vi "Teleop.vi"(0 "Call Context":T9) -> (6 "SubState 3":T4, 9 "SubState 4":T8, 11 "Loop 3 Data":T3, 14 "SubState 0":T4=enum."driver control", 15 "Loop 1 Data":T6, 16 "Loop 0 Data":T7, 17 "SubState 1":T4, 18 "Loop 2 Data":T5, 19 "SubState 2":T4)   [LabVIEW 2013]
uses:
  typedefs/State Machine/subStates.ctl
  <vilib>/Rock Robotics/WPI/DriverStation/WPI_DriverStationDerivedRobotMode.ctl
  typedefs/State Machine/singleUseSubstate.ctl
  typedefs/Loop Datatypes/Loop 0 Datatype.ctl
  typedefs/Loop Datatypes/Loop 1 Datatype.ctl
  typedefs/Loop Datatypes/Loop 2 Datatype.ctl
  typedefs/Loop Datatypes/Loop 3 Datatype.ctl
  <vilib>/Rock Robotics/WPI/Joystick/WPI_JoystickDevRef.ctl
  <vilib>/Rock Robotics/WPI/Joystick/WPI_JoystickDeviceEnum.ctl
  typedefs/fg_typedef.ctl
  typedefs/Vision/vision enable.ctl
  <vilib>/Rock Robotics/WPI/Joystick/WPI_JoystickGetSetRefNum.vi
panel:
  out "FDC":bool
  out "JS3":T1
  out "Drive to DC":bool
  out "JS1":T1
  out "JS2":T1
  out "Exit Value":i32=-1
  # "Loop Data and Substates"
  # "Drive Loop"
  # "State Machine Master Loop"
  # "Pickup/Passing Belts Loop"
  # "Pickup/Passing Arm Loop"
  # "Pneumatics Loop"
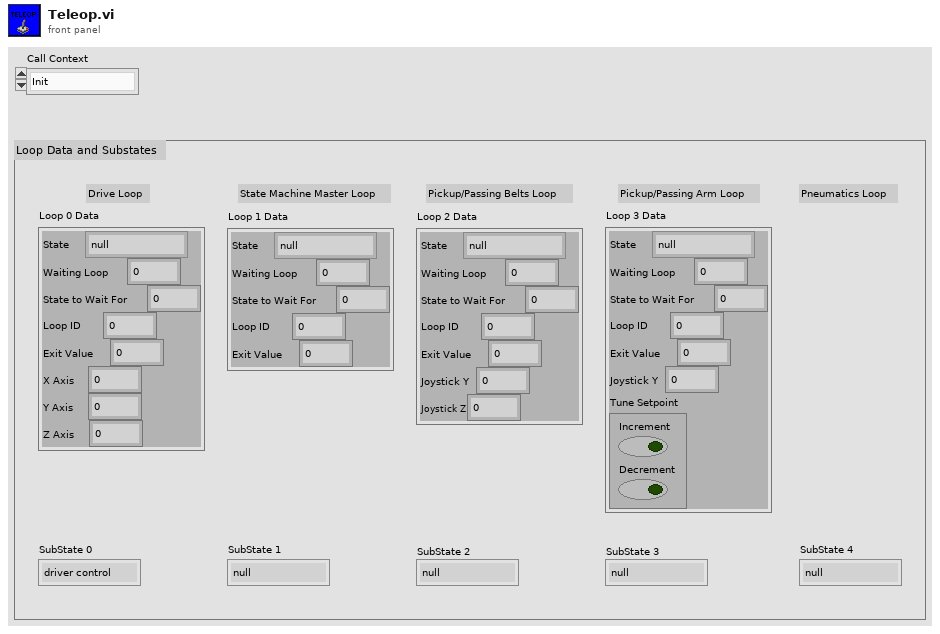
[diagram p1: front panel]
types:
  T1 = typedef "WPI_JoystickDevRef.ctl" = cluster{"Device":T2}
  T2 = typedef "WPI_JoystickDeviceEnum.ctl" = enum16{"USB 1", "USB 2", "USB 3", "USB 4", "Kinect 1", "Kinect 2"}
  T3 = typedef "Loop 3 Datatype.ctl" = cluster{"State":T4, "Waiting Loop":i32, "State to Wait For":i32, "Loop ID":i32, "Exit Value":i32, "Joystick Y":dbl, "Tune Setpoint":cluster{"Increment":bool, "Decrement":bool}}
  T4 = typedef "subStates.ctl" = enum16{"null", "wait", "driver control", "auto", "manual override", "hold position", "rotate", "pickup", "pass", "recover pass", "load", "goto shoot", "shoot high goal", "shoot low goal", "cancel arm", "cancel shooter", "end", "test"}
  T5 = typedef "Loop 2 Datatype.ctl" = cluster{"State":T4, "Waiting Loop":i32, "State to Wait For":i32, "Loop ID":i32, "Exit Value":i32, "Joystick Y":dbl, "Joystick Z":dbl}
  T6 = typedef "Loop 1 Datatype.ctl" = cluster{"State":T4, "Waiting Loop":i32, "State to Wait For":i32, "Loop ID":i32, "Exit Value":i32}
  T7 = typedef "Loop 0 Datatype.ctl" = cluster{"State":T4, "Waiting Loop":i32, "State to Wait For":i32, "Loop ID":i32, "Exit Value":i32, "X Axis":dbl, "Y Axis":dbl, "Z Axis":dbl}
  T8 = typedef "singleUseSubstate.ctl" = enum16{"null", "wait", "shift high", "shift low", "extend shooter", "retract shooter", "latch", "unlatch", "end"}
  T9 = typedef "WPI_DriverStationDerivedRobotMode.ctl" = enum16{"Init", "Execute", "Stop"}
  T10 = typedef "fg_typedef.ctl" = enum16{"Get", "Set"}
  T11 = cluster{"axis 1 (x)":dbl, "axis 2 (y)":dbl, "axis 3 (throttle)":dbl, "axis 4":dbl, "axis 5":dbl, "axis 6":dbl}
  T12 = typedef "WPI_EncoderDevRef.ctl" = cluster{"DevStatus":errorcluster, "EncoderIndex":T13, "CounterIndex":T14, "DistancePerCount":dbl, "Decoding Type":T15}
  T13 = typedef "FPGA_EncoderIdx.ctl" = enum8{"Enc 0", "Enc 1", "Enc 2", "Enc 3", "Invalid"}
  T14 = typedef "FPGA_CounterCtrSystemIndex.ctl" = enum8{"Ctr 0", "Ctr 1", "Ctr 2", "Ctr 3", "Ctr 4", "Ctr 5", "Ctr 6", "Ctr 7", "Invalid"}
  T15 = typedef "WPI_EncoderType.ctl" = enum16{"1x", "2x", "4x"}
  T16 = typedef "vision enable.ctl" = enum16{"Enable", "Disable", "Stop"}
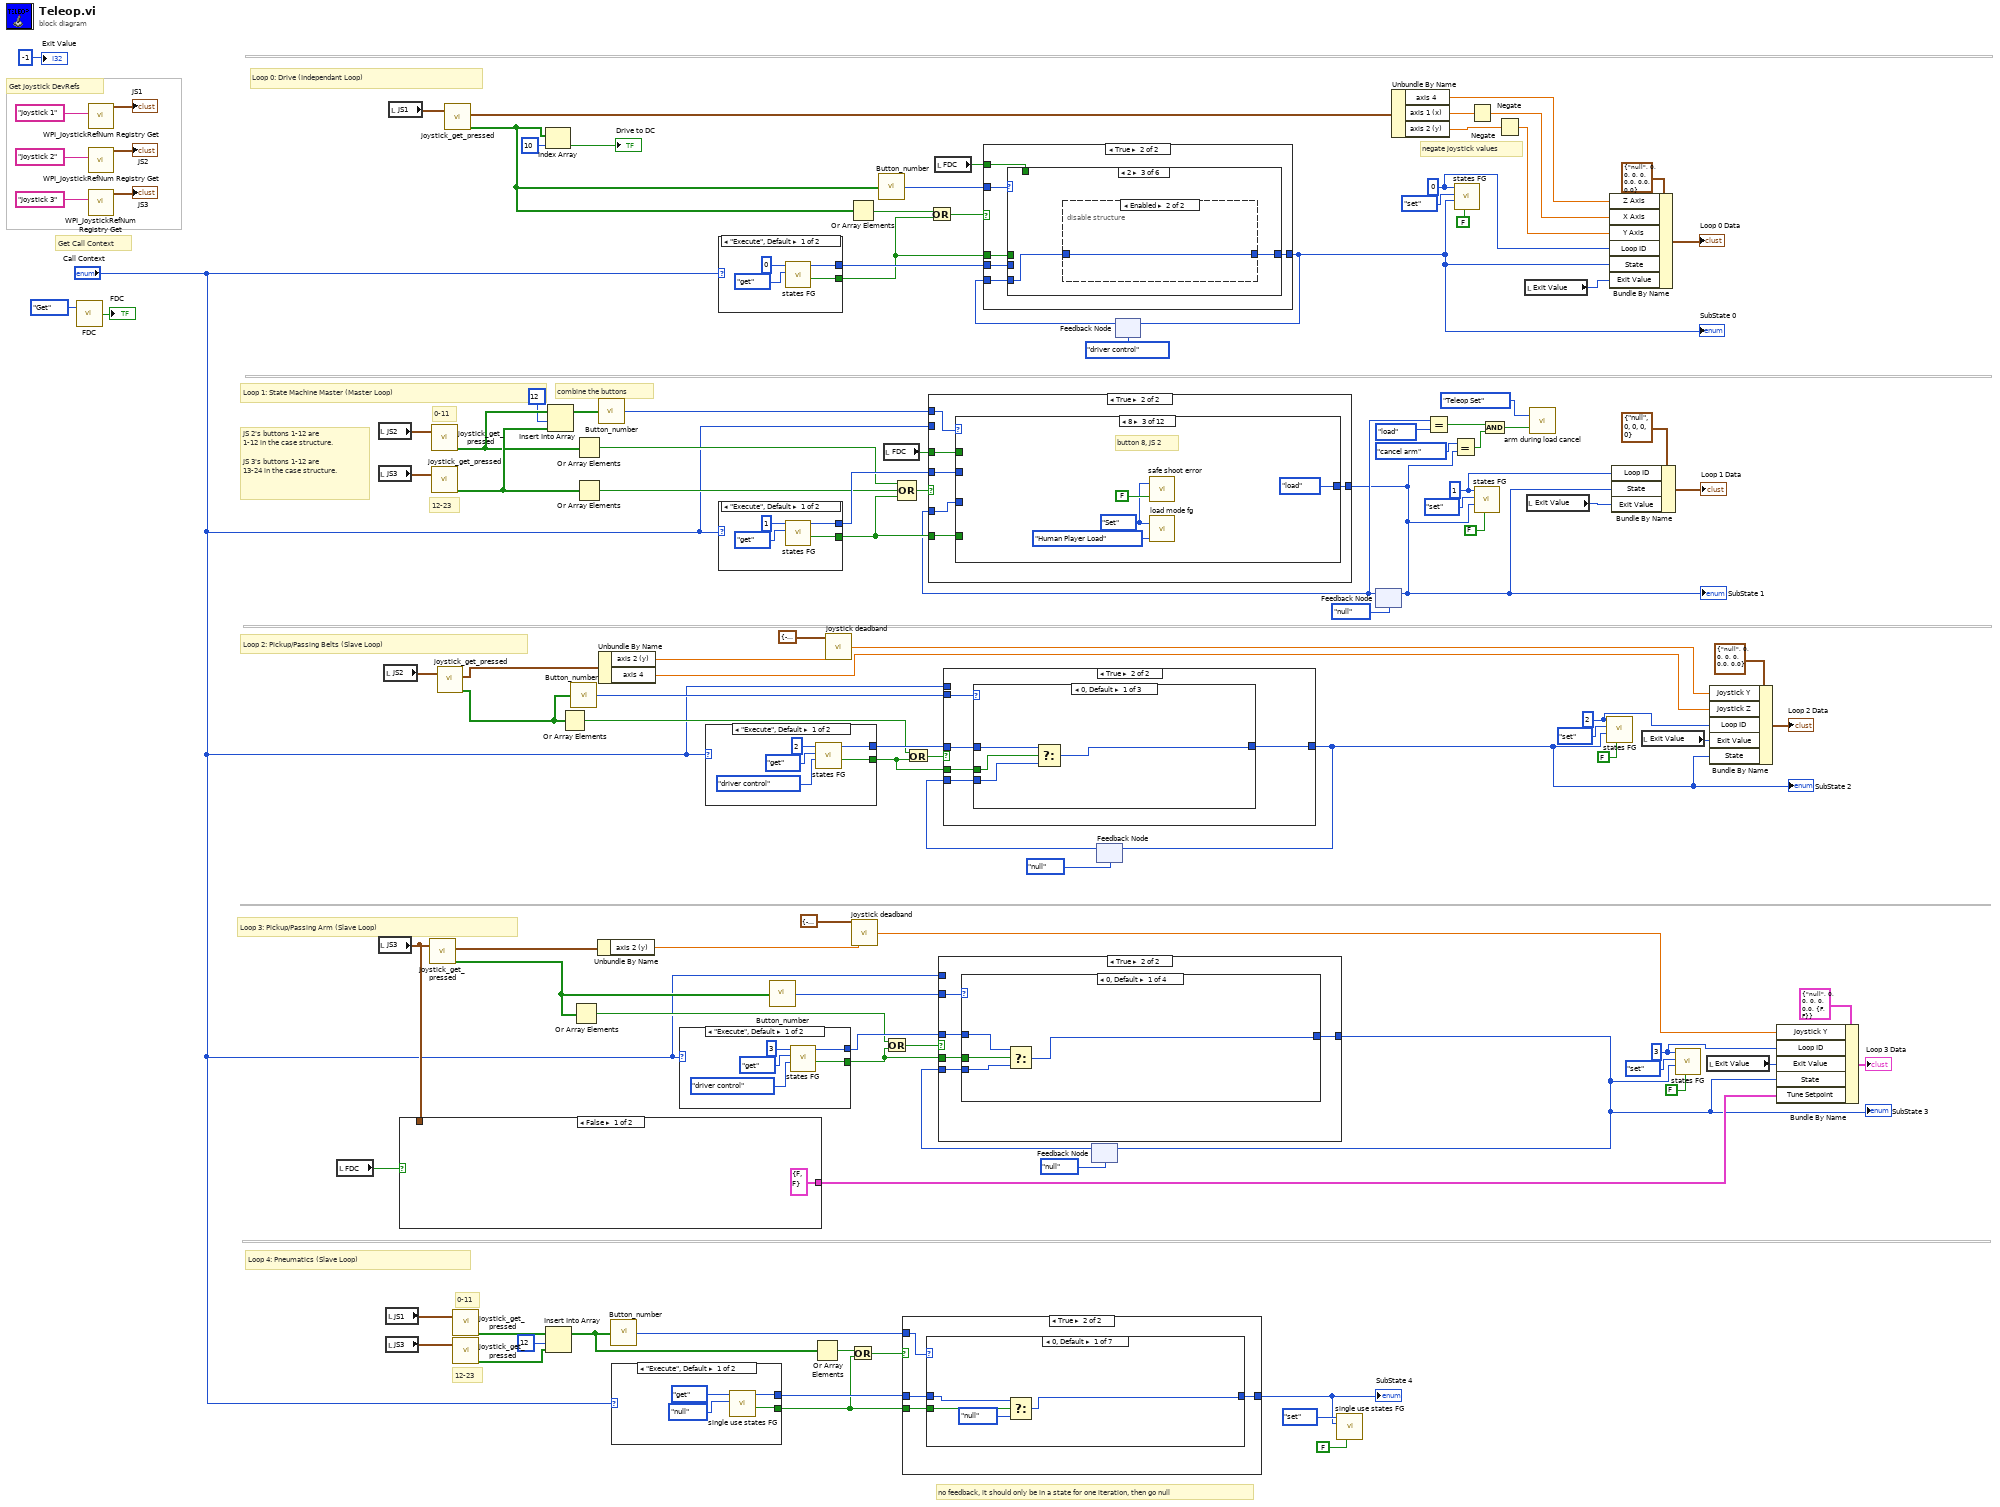
[diagram p0: block diagram]
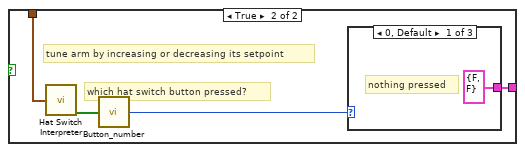
[diagram p2: hidden frame]
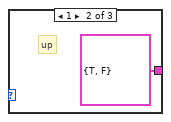
[diagram p3: hidden frame]
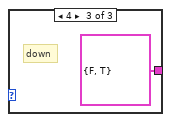
[diagram p4: hidden frame]
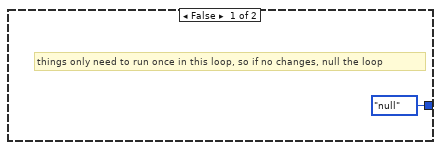
[diagram p5: hidden frame]
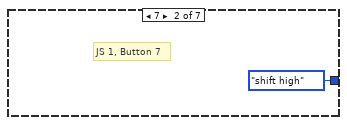
[diagram p6: hidden frame]
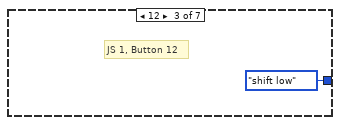
[diagram p7: hidden frame]
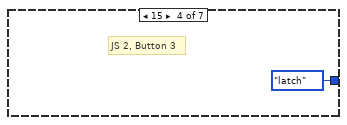
[diagram p8: hidden frame]
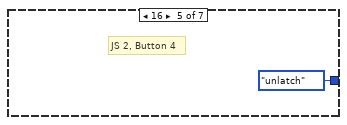
[diagram p9: hidden frame]
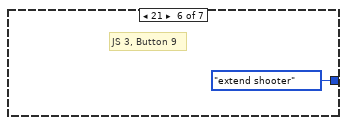
[diagram p10: hidden frame]
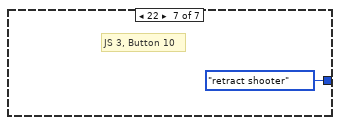
[diagram p11: hidden frame]
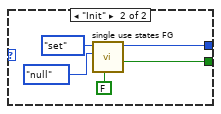
[diagram p12: hidden frame]
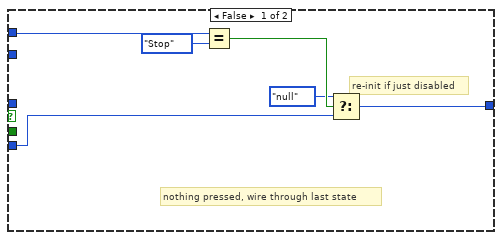
[diagram p13: hidden frame]
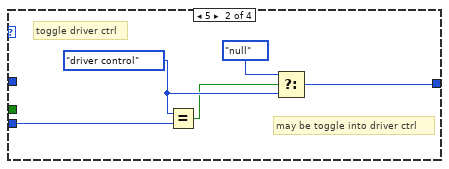
[diagram p14: hidden frame]
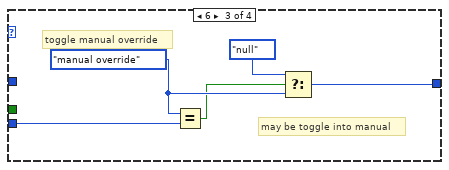
[diagram p15: hidden frame]
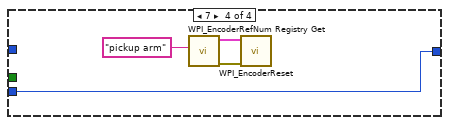
[diagram p16: hidden frame]
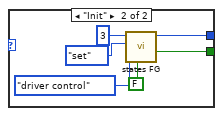
[diagram p17: hidden frame]
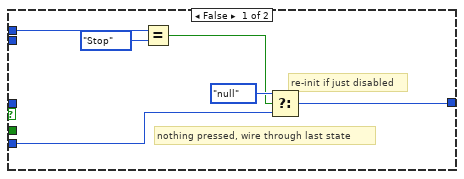
[diagram p18: hidden frame]
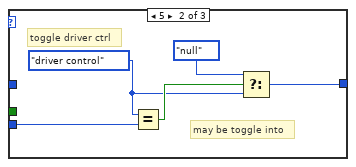
[diagram p19: hidden frame]
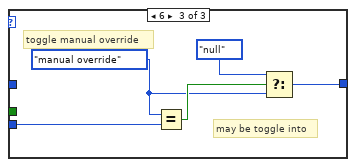
[diagram p20: hidden frame]
diagram:
  w93 = 3 ("Loop ID")
  w94 = 2 ("Loop ID")
  w103 = 1 ("Loop ID")
  w105 = 0 ("Loop ID")
  # "12-23"
  # "0-11"
  # "no feedback, it should only be in a state for one iteration, then go null"
  # "JS 2's buttons 1-12 are\n1-12 in the case structure.\n\nJS 3's buttons 1-12 are\n13-24 in the case structure."
  # "combine the buttons"
  # "12-23"
  # "0-11"
  # "negate joystick values"
  # "Get Call Context"
  # "Get Joystick DevRefs"
  # "Loop 3: Pickup/Passing Arm (Slave Loop)"
  # "Loop 4: Pneumatics (Slave Loop)"
  # "Loop 2: Pickup/Passing Belts (Slave Loop)"
  # "Loop 1: State Machine Master (Master Loop)"
  # "Loop 0: Drive (Independant Loop)"
  n1 = call "FDC.vi"("Menu"=fg_typedef."Get") -> ("FDC"=→"FDC":bool)  [unwired: 1 in]
  n2 = call <vilib>:"WPI_JoystickRefNum Registry Get.vi"("refnum name"="Joystick 1") -> ("JoystickDevRef"=→"JS1":T1)  [unwired: 9 in, 1 out]
  n3 = call <vilib>:"WPI_JoystickRefNum Registry Get.vi"("refnum name"="Joystick 2") -> ("JoystickDevRef"=→"JS2":T1)  [unwired: 9 in, 1 out]
  n4 = call <vilib>:"WPI_JoystickRefNum Registry Get.vi"("refnum name"="Joystick 3") -> ("JoystickDevRef"=→"JS3":T1)  [unwired: 9 in, 1 out]
  n5 = local read "FDC"() -> (w1:bool)
  n6 = local read "JS2"() -> (w73:T1)
  n7 = local read "JS3"() -> (w31:T1)
  n8 = local read "JS3"() -> (w40:T1)
  n9 = local read "JS2"() -> (w51:T1)
  n10 = local read "JS1"() -> (w54:T1)
  n11 = local read "JS3"() -> (w16:T1)
  n12 = local read "JS1"() -> (w74:T1)
  n13 = case shown="False" w1 {
    tunnel: w40 -> [_ w125]
    tunnel: [cluster{"Increment":bool, "Decrement":bool} {"Increment"=FALSE, "Decrement"=FALSE} w122] -> w38
    frame False {
    }
    frame True {
      # "tune arm by increasing or decreasing its setpoint"
      # "which hat switch button pressed?"
      n14 = call "Hat Switch Interpreter.vi"("JoystickDevRef"=w125) -> ("Buttons"=w124:bool[])  [unwired: 4 out]
      n15 = call "Button_number.vi"("Button Array"=w124) -> ("Button Pressed"=w123:i32)
      n16 = case shown="0, Default" w123 {
        tunnel: [cluster{"Increment":bool, "Decrement":bool} {"Increment"=FALSE, "Decrement"=FALSE} cluster{"Increment":bool, "Decrement":bool} {"Increment"=TRUE, "Decrement"=FALSE} cluster{"Increment":bool, "Decrement":bool} {"Increment"=FALSE, "Decrement"=TRUE}] -> w122
        frame 0, Default {
          # "nothing pressed"
        }
        frame 1 {
          # "up"
        }
        frame 4 {
          # "down"
        }
      }
    }
  }
  n17 = call "joystick_get_pressed.vi"("JoystickDevRef 2"=w40) -> ("Axes"=w63:T11, "Buttons Pressed?"=w7:bool[])  [unwired: 1 in, 2 out]
  n18 = call "joystick_get_pressed.vi"("JoystickDevRef 2"=w73) -> ("Buttons Pressed?"=w27:bool[])  [unwired: 1 in, 3 out]
  n19 = call "joystick_get_pressed.vi"("JoystickDevRef 2"=w31) -> ("Buttons Pressed?"=w28:bool[])  [unwired: 1 in, 3 out]
  n20 = call "joystick_get_pressed.vi"("JoystickDevRef 2"=w51) -> ("Axes"=w43:T11, "Buttons Pressed?"=w8:bool[])  [unwired: 1 in, 2 out]
  n21 = call "joystick_get_pressed.vi"("JoystickDevRef 2"=w74) -> ("Axes"=w78:T11, "Buttons Pressed?"=w56:bool[])  [unwired: 1 in, 2 out]
  n22 = call "joystick_get_pressed.vi"("JoystickDevRef 2"=w54) -> ("Buttons Pressed?"=w13:bool[])  [unwired: 1 in, 3 out]
  n23 = call "joystick_get_pressed.vi"("JoystickDevRef 2"=w16) -> ("Buttons Pressed?"=w14:bool[])  [unwired: 1 in, 3 out]
  n24 = Index Array(array=w56, index=10) -> (element=→"Drive to DC":bool)
  n25 = Insert Into Array(array=w13, index=12, new element=w14) -> (w12:bool[])
  n26 = Insert Into Array(array=w27, index=12, new element=w28) -> (w25:bool[])
  n27 = Or Array Elements(Boolean array=w8) -> (logical OR=w50:bool)
  n28 = call "Button_number.vi"("Button Array"=w8) -> ("Button Pressed"=w49:i32)
  n29 = Or Array Elements(Boolean array=w7) -> (logical OR=w62:bool)
  n30 = Or Array Elements(Boolean array=w27) -> (logical OR=w30:bool)
  n31 = Or Array Elements(Boolean array=w28) -> (logical OR=w29:bool)
  n32 = Unbundle By Name(w63) -> ("axis 2 (y)"=w59:dbl)
  n33 = call "Button_number.vi"("Button Array"=w25) -> ("Button Pressed"=w67:i32)
  n34 = Unbundle By Name(w43) -> ("axis 2 (y)"=w45:dbl, "axis 4"=w41:dbl)
  n35 = call "Button_number.vi"("Button Array"=w12) -> ("Button Pressed"=w33:i32)
  n36 = case shown="\"Execute\", Default" "Call Context" {
    tunnel: [w131 w134] -> w32
    tunnel: [w132 w133] -> w44
    frame "Execute", Default {
      n37 = call "single use states FG.vi"("substate"=singleUseSubstate."null" ("Enum"), "menu (get)"=enum16{"set", "get"}."get") -> ("exit out"=w131:bool, "substate out"=w132:T8)  [unwired: 6 in, 2 out]
    }
    frame "Init" {
      n38 = call "single use states FG.vi"("exit in"=FALSE, "substate"=singleUseSubstate."null", "menu (get)"=enum16{"set", "get"}."set") -> ("exit out"=w134:bool, "substate out"=w133:T8)  [unwired: 5 in, 2 out]
    }
  }
  n39 = case shown="\"Execute\", Default" "Call Context" {
    tunnel: [w140 w146] -> w60
    tunnel: [w138 w143] -> w91
    frame "Execute", Default {
      n40 = call "states FG.vi"("subState in"=subStates."driver control", "menu (get)"=enum16{"set", "get"}."get", "Loop ID"=3) -> ("exit out"=w140:bool, "subState out"=w138:T4)  [unwired: 5 in, 2 out]
    }
    frame "Init" {
      n41 = call "states FG.vi"("exit in"=FALSE, "subState in"=subStates."driver control", "menu (get)"=enum16{"set", "get"}."set", "Loop ID"=3) -> ("exit out"=w146:bool, "subState out"=w143:T4)  [unwired: 4 in, 2 out]
    }
  }
  n42 = case shown="\"Execute\", Default" "Call Context" {
    tunnel: [w151 w157] -> w65
    tunnel: [w149 w154] -> w109
    frame "Execute", Default {
      n43 = call "states FG.vi"("subState in"=subStates."driver control", "menu (get)"=enum16{"set", "get"}."get", "Loop ID"=2) -> ("exit out"=w151:bool, "subState out"=w149:T4)  [unwired: 5 in, 2 out]
    }
    frame "Init" {
      n44 = call "states FG.vi"("exit in"=FALSE, "subState in"=subStates."driver control", "menu (get)"=enum16{"set", "get"}."set", "Loop ID"=2) -> ("exit out"=w157:bool, "subState out"=w154:T4)  [unwired: 4 in, 2 out]
    }
  }
  n45 = case shown="\"Execute\", Default" "Call Context" {
    tunnel: [w161 w166] -> w71
    tunnel: [w160 w164] -> w108
    frame "Execute", Default {
      n46 = call "states FG.vi"("menu (get)"=enum16{"set", "get"}."get", "Loop ID"=0) -> ("exit out"=w161:bool, "subState out"=w160:T4)  [unwired: 6 in, 2 out]
    }
    frame "Init" {
      n47 = call "states FG.vi"("exit in"=FALSE, "menu (get)"=enum16{"set", "get"}."set", "Loop ID"=0) -> ("exit out"=w166:bool, "subState out"=w164:T4)  [unwired: 5 in, 2 out]
    }
  }
  n48 = case shown="\"Execute\", Default" "Call Context" {
    tunnel: [w170 w175] -> w68
    tunnel: [w169 w173] -> w107
    frame "Execute", Default {
      n49 = call "states FG.vi"("menu (get)"=enum16{"set", "get"}."get", "Loop ID"=1) -> ("exit out"=w170:bool, "subState out"=w169:T4)  [unwired: 6 in, 2 out]
    }
    frame "Init" {
      n50 = call "states FG.vi"("exit in"=FALSE, "menu (get)"=enum16{"set", "get"}."set", "Loop ID"=1) -> ("exit out"=w175:bool, "subState out"=w173:T4)  [unwired: 5 in, 2 out]
    }
  }
  n51 = call "Button_number.vi"("Button Array"=w7) -> ("Button Pressed"=w61:i32)
  n52 = Or Array Elements(Boolean array=w12) -> (logical OR=w34:bool)
  n53 = call "joystick deadband.vi"("Joystick In"=w45, "Deadband Range"=cluster{"Deadband Min":dbl, "Deadband Max":dbl} {"Deadband Min"=-0.09, "Deadband Max"=0.09}) -> ("Joystick Out"=w42:dbl)  [unwired: 4 in]
  n54 = Or Array Elements(Boolean array=w56) -> (logical OR=w72:bool)
  n55 = Or(x=w34, y=w32) -> (x .or. y?=w35:bool)
  n56 = call "joystick deadband.vi"("Joystick In"=w59, "Deadband Range"=cluster{"Deadband Min":dbl, "Deadband Max":dbl} {"Deadband Min"=-0.09, "Deadband Max"=0.09}) -> ("Joystick Out"=w39:dbl)  [unwired: 4 in]
  n57 = call "Button_number.vi"("Button Array"=w56) -> ("Button Pressed"=w77:i32)
  n58 = local read "FDC"() -> (w2:bool)
  n59 = Or(x=w62, y=w60) -> (x .or. y?=w64:bool)
  n60 = Compound Arithmetic op=OR(w30, w29, w68) -> (w69:bool)
  n61 = case shown="True" w35 {
    tunnel: [singleUseSubstate."null" ("Enum") w179] -> w10
    tunnel: w44 -> [_ w180]
    tunnel: w33 -> [_ w181]
    tunnel: w32 -> [_ w182]
    frame False {
      # "things only need to run once in this loop, so if no changes, null the loop"
    }
    frame True {
      n62 = case shown="0, Default" w181 {
        tunnel: w182 -> [w186 _ _ _ _ _ _]
        tunnel: w180 -> [w185 _ _ _ _ _ _]
        tunnel: [w184 singleUseSubstate."shift high" ("Enum") singleUseSubstate."shift low" ("Enum") singleUseSubstate."latch" ("Enum") singleUseSubstate."unlatch" ("Enum") singleUseSubstate."extend shooter" ("Enum") singleUseSubstate."retract shooter" ("Enum")] -> w179
        frame 0, Default {
          n63 = Select(t=w185, s=w186, f=singleUseSubstate."null") -> (s? t:f=w184:T8)
        }
        frame 7 {
          # "JS 1, Button 7"
        }
        frame 12 {
          # "JS 1, Button 12"
        }
        frame 15 {
          # "JS 2, Button 3"
        }
        frame 16 {
          # "JS 2, Button 4"
        }
        frame 21 {
          # "JS 3, Button 9"
        }
        frame 22 {
          # "JS 3, Button 10"
        }
      }
    }
  }
  "SubState 4" <- w10
  n64 = Or(x=w50, y=w65) -> (x .or. y?=w66:bool)
  n65 = Or(x=w72, y=w71) -> (x .or. y?=w70:bool)
  n66 = local read "FDC"() -> (w3:bool)
  n67 = feedback #1(subStates."null" ("Drive SubState")) -> (w88:T4)
  n68 = case shown="True" w64 {
    tunnel: w88 -> [w195 w199]
    tunnel: [w194 w200] -> w37
    tunnel: w91 -> [_ w201]
    tunnel: w61 -> [_ w203]
    tunnel: w60 -> [_ w202]
    tunnel: "Call Context" -> [w193 _]
    frame False {
      # "nothing pressed, wire through last state"
      # "re-init if just disabled"
      n69 = Equal?(x=w193, y=WPI_DriverStationDerivedRobotMode."Stop") -> (x = y?=w197:bool)
      n70 = Select(t=subStates."null", s=w197, f=w195) -> (s? t:f=w194:T4)
    }
    frame True {
      n71 = case shown="0, Default" w203 {
        tunnel: w202 -> [w207 _ _ _]
        tunnel: w199 -> [w206 w208 w213 w221]
        tunnel: w201 -> [w205 _ _ _]
        tunnel: [w204 w209 w214 w221] -> w200
        frame 0, Default {
          n72 = Select(t=w205, s=w207, f=w206) -> (s? t:f=w204:T4)
        }
        frame 5 {
          w211 = subStates."driver control" ("Drive SubState")
          # "may be toggle into driver ctrl"
          # "toggle driver ctrl"
          n73 = Equal?(x=w211, y=w208) -> (x = y?=w210:bool)
          n74 = Select(t=subStates."null", s=w210, f=w211) -> (s? t:f=w209:T4)
        }
        frame 6 {
          w217 = subStates."manual override" ("Drive SubState")
          # "may be toggle into manual"
          # "toggle manual override"
          n75 = Equal?(x=w217, y=w213) -> (x = y?=w215:bool)
          n76 = Select(t=subStates."null", s=w215, f=w217) -> (s? t:f=w214:T4)
        }
        frame 7 {
          n77 = call <vilib>:"WPI_EncoderRefNum Registry Get.vi"("refnum name"="pickup arm") -> ("error out"=w219:errorcluster, "EncoderDevRef"=w218:T12)  [unwired: 9 in]
          n78 = call <vilib>:"WPI_EncoderReset.vi"("error in (no error)"=w219, "EncoderDevRef"=w218) -> ()  [unwired: 8 in, 2 out]
        }
      }
    }
  }
  "SubState 3" <- w37
  n79 = feedback-in #1(w37) -> ()
  n80 = feedback #2(subStates."null" ("Drive SubState")) -> (w112:T4)
  n81 = case shown="True" w66 {
    tunnel: w112 -> [w223 w229]
    tunnel: [w222 w228] -> w36
    tunnel: w109 -> [_ w230]
    tunnel: w49 -> [_ w232]
    tunnel: w65 -> [_ w231]
    tunnel: "Call Context" -> [w224 _]
    frame False {
      # "re-init if just disabled"
      # "nothing pressed, wire through last state"
      n82 = Equal?(x=w224, y=WPI_DriverStationDerivedRobotMode."Stop") -> (x = y?=w226:bool)
      n83 = Select(t=subStates."null", s=w226, f=w223) -> (s? t:f=w222:T4)
    }
    frame True {
      n84 = case shown="0, Default" w232 {
        tunnel: w231 -> [w236 _ _]
        tunnel: w230 -> [w235 _ _]
        tunnel: w229 -> [w234 w241 w243]
        tunnel: [w233 w237 w242] -> w228
        frame 0, Default {
          n85 = Select(t=w235, s=w236, f=w234) -> (s? t:f=w233:T4)
        }
        frame 5 {
          w239 = subStates."driver control" ("Drive SubState")
          # "may be toggle into"
          # "toggle driver ctrl"
          n86 = Equal?(x=w239, y=w241) -> (x = y?=w240:bool)
          n87 = Select(t=subStates."null", s=w240, f=w239) -> (s? t:f=w237:T4)
        }
        frame 6 {
          w244 = subStates."manual override" ("Drive SubState")
          # "may be toggle into"
          # "toggle manual override"
          n88 = Equal?(x=w244, y=w243) -> (x = y?=w246:bool)
          n89 = Select(t=subStates."null", s=w246, f=w244) -> (s? t:f=w242:T4)
        }
      }
    }
  }
  "SubState 2" <- w36
  n90 = feedback-in #2(w36) -> ()
  n91 = feedback #3(subStates."driver control" ("Drive SubState")) -> (w114:T4)
  n92 = case shown="True" w70 {
    tunnel: w114 -> [w247 w250]
    tunnel: [w247 w249] -> w53
    tunnel: w108 -> [_ w251]
    tunnel: w77 -> [_ w253]
    tunnel: w71 -> [_ w252]
    tunnel: w3 -> [_ w248]
    frame False {
      # "keep current state, no change necessary"
    }
    frame True {
      n93 = case shown="2" w253 {
        tunnel: w252 -> [w257 _ _ _ _ _]
        tunnel: w251 -> [w256 _ _ _ _ _]
        tunnel: w250 -> [w255 w262 w263 w268 w276 _]
        tunnel: [w254 w258 w264 w268 w277 subStates."driver control" ("Drive SubState")] -> w249
        tunnel: w248 -> [_ _ _ w267 _ _]
        frame 0, Default {
          n94 = Select(t=w256, s=w257, f=w255) -> (s? t:f=w254:T4)
        }
        frame 1 {
          w259 = subStates."hold position" ("x")
          # "button 1, hold position toggle"
          n95 = Equal?(x=w259, y=w262) -> (x = y?=w261:bool)
          n96 = Select(t=subStates."driver control" ("Drive SubState"), s=w261, f=w259) -> (s? t:f=w258:T4)
        }
        frame 2 {
          n97 = disable-structure shown="Enabled" {
            disable-tunnel: [subStates."manual override" ("Drive SubState") w266] -> w264
            disable-tunnel: w263 -> [_ w266]
            frame Disabled {
            }
            frame Enabled {
            }
          }
        }
        frame 8 {
          n98 = case shown="True" w267 {
            frame False {
            }
            frame True {
              w271 = vision_enable."Enable" ("y")
              # "toggle vision"
              n99 = call "vision_fg.vi"("Menu"=fg_typedef."Get") -> ("State Out"=w273:T16)  [unwired: 2 in, 1 out]
              n100 = Equal?(x=w273, y=w271) -> (x = y?=w272:bool)
              n101 = Select(t=vision_enable."Disable" ("y"), s=w272, f=w271) -> (s? t:f=w269:T16)
              n102 = call "vision_fg.vi"("Action"=w269, "Menu"=fg_typedef."Set") -> ()  [unwired: 1 in, 2 out]
            }
          }
        }
        frame 10 {
          n103 = disable-structure shown="Enabled" {
            disable-tunnel: [subStates."goto shoot" ("Drive SubState") w281] -> w277
            disable-tunnel: w276 -> [_ w281]
            frame Disabled {
              # "go to shoot location"
              n104 = call "vision_fg.vi"("Action"=vision_enable."Enable", "Menu"=fg_typedef."Set") -> ()  [unwired: 1 in, 2 out]
            }
            frame Enabled {
            }
          }
        }
        frame 11 {
          # "put robot drive in driver control"
          n105 = call "vision_fg.vi"("Action"=vision_enable."Disable", "Menu"=fg_typedef."Set") -> ()  [unwired: 1 in, 2 out]
        }
      }
    }
  }
  "SubState 0" <- w53
  n106 = feedback-in #3(w53) -> ()
  n107 = call "single use states FG.vi"("exit in"=FALSE, "substate"=w10, "menu (get)"=enum16{"set", "get"}."set") -> ()  [unwired: 5 in, 4 out]
  n108 = feedback #4(subStates."null" ("Drive SubState")) -> (w22:T4)
  n109 = case shown="True" w69 {
    tunnel: w22 -> [w287 w295]
    tunnel: [w285 w294] -> w19
    tunnel: w107 -> [_ w296]
    tunnel: w67 -> [_ w293]
    tunnel: w68 -> [_ w292]
    tunnel: "Call Context" -> [w290 _]
    tunnel: w2 -> [_ w291]
    frame False {
      # "re-init if just disabled"
      # "nothing pressed here, move along (wire through the previous state)"
      n110 = Equal?(x=w290, y=WPI_DriverStationDerivedRobotMode."Stop") -> (x = y?=w288:bool)
      n111 = Select(t=subStates."null", s=w288, f=w287) -> (s? t:f=w285:T4)
    }
    frame True {
      n112 = case shown="8" w293 {
        tunnel: w296 -> [w300 _ _ _ _ _ _ _ _ _ _ _]
        tunnel: w295 -> [w299 _ _ w306 w311 w316 w321 _ w327 _ w336 w341]
        tunnel: [w298 subStates."null" ("Drive SubState") subStates."load" ("Drive SubState") w308 w313 w318 w323 subStates."shoot high goal" ("Drive SubState") w332 subStates."manual override" ("Drive SubState") w338 w343] -> w294
        tunnel: w292 -> [w297 _ _ _ _ _ _ _ _ _ _ _]
        tunnel: w291 -> [_ _ _ w307 w312 w317 w322 _ w328 _ w337 w342]
        frame 0, Default {
          n113 = Select(t=w300, s=w297, f=w299) -> (s? t:f=w298:T4)
        }
        frame 2 {
          # "null the state machine"
          # "JS 2 button 2"
        }
        frame 8 {
          w302 = fg_typedef."Set" ("Menu")
          # "button 8, JS 2"
          n114 = call "safe shoot error.vi"("Can Shoot Safely?"=FALSE, "Menu"=w302) -> ()  [unwired: 1 out]
          n115 = call "load mode fg.vi"("Load Mode"=enum16{"Feild Load", "Human Player Load"}."Human Player Load", "Menu"=w302) -> ()  [unwired: 1 out]
        }
        frame 9 {
          # "button 9, JS 2"
          n116 = case shown="True" w307 {
            tunnel: [w309 subStates."cancel arm" ("Drive SubState")] -> w308
            tunnel: w306 -> [w309 _]
            frame False {
            }
            frame True {
            }
          }
        }
        frame 10 {
          # "button 10, JS2, recover pass"
          n117 = case shown="True" w312 {
            tunnel: [w314 subStates."recover pass" ("Drive SubState")] -> w313
            tunnel: w311 -> [w314 _]
            frame False {
            }
            frame True {
            }
          }
        }
        frame 11 {
          # "button 11, JS 2"
          n118 = case shown="True" w317 {
            tunnel: [w319 subStates."pickup" ("Drive SubState")] -> w318
            tunnel: w316 -> [w319 _]
            frame False {
            }
            frame True {
            }
          }
        }
        frame 12 {
          # "button 12, JS 2"
          n119 = case shown="True" w322 {
            tunnel: [w324 subStates."pass" ("Drive SubState")] -> w323
            tunnel: w321 -> [w324 _]
            frame False {
            }
            frame True {
            }
          }
        }
        frame 13 {
          # "button 1, JS 3"
        }
        frame 14 {
          w330 = fg_typedef."Set" ("Menu")
          # "button 2, JS 3"
          n120 = call "safe shoot error.vi"("Can Shoot Safely?"=FALSE, "Menu"=w330) -> ()  [unwired: 1 out]
          n121 = call "load mode fg.vi"("Load Mode"=enum16{"Feild Load", "Human Player Load"}."Feild Load", "Menu"=w330) -> ()  [unwired: 1 out]
          n122 = case shown="True" w328 {
            tunnel: [w333 subStates."load" ("Drive SubState")] -> w332
            tunnel: w327 -> [w333 _]
            frame False {
            }
            frame True {
            }
          }
        }
        frame 20 {
          # "manual shoot"
          # "button 8, JS 3"
        }
        frame 23 {
          # "button 11, JS 3"
          n123 = case shown="False" w337 {
            tunnel: [w339 subStates."shoot low goal" ("Drive SubState")] -> w338
            tunnel: w336 -> [w339 _]
            frame False {
            }
            frame True {
            }
          }
        }
        frame 24 {
          # "button 12, JS 3"
          n124 = case shown="True" w342 {
            tunnel: [w344 subStates."cancel shooter" ("Drive SubState")] -> w343
            tunnel: w341 -> [w344 _]
            frame False {
            }
            frame True {
            }
          }
        }
      }
    }
  }
  "SubState 1" <- w19
  n125 = feedback-in #4(w19) -> ()
  n126 = Unbundle By Name(w78) -> ("axis 4"=w57:dbl, "axis 1 (x)"=w82:dbl, "axis 2 (y)"=w81:dbl)
  n127 = Equal?(x=w22, y=subStates."load") -> (x = y?=w20:bool)
  n128 = Equal?(x=subStates."cancel arm" ("y"), y=w19) -> (x = y?=w21:bool)
  n129 = call "states FG.vi"("exit in"=FALSE, "subState in"=w53, "menu (get)"=enum16{"set", "get"}."set", "Loop ID"=w105) -> ()  [unwired: 4 in, 4 out]
  n130 = Negate(x=w82) -> (-x=w80:dbl)
  n131 = call "states FG.vi"("exit in"=FALSE, "subState in"=w19, "menu (get)"=enum16{"set", "get"}."set", "Loop ID"=w103) -> ()  [unwired: 4 in, 4 out]
  n132 = And(x=w20, y=w21) -> (x .and. y?=w18:bool)
  n133 = Negate(x=w81) -> (-x=w79:dbl)
  n134 = local read "Exit Value"() -> (w101:i32)
  n135 = local read "Exit Value"() -> (w100:i32)
  n136 = call "arm during load cancel.vi"("Arm Canceled During Load?"=w18, "Mode"=enum16{"Get", "Set", "Teleop Set"}."Teleop Set") -> ()  [unwired: 1 out]
  n137 = call "states FG.vi"("exit in"=FALSE, "subState in"=w36, "menu (get)"=enum16{"set", "get"}."set", "Loop ID"=w94) -> ()  [unwired: 4 in, 4 out]
  n138 = Bundle By Name(cluster=T7 {"State"=enum."null", "Waiting Loop"=0, "State to Wait For"=0, "Loop ID"=0, "Exit Value"=0, "X Axis"=0.0, "Y Axis"=0.0, "Z Axis"=0.0} ("Cluster"), "Z Axis"=w57, "X Axis"=w80, "Y Axis"=w79, "Loop ID"=w105, "State"=w53, "Exit Value"=w101) -> (→"Loop 0 Data":T7)
  n139 = Bundle By Name(cluster=T6 {"State"=enum."null", "Waiting Loop"=0, "State to Wait For"=0, "Loop ID"=0, "Exit Value"=0} ("Cluster"), "Loop ID"=w103, "State"=w19, "Exit Value"=w100) -> (→"Loop 1 Data":T6)
  n140 = local read "Exit Value"() -> (w95:i32)
  n141 = call "states FG.vi"("exit in"=FALSE, "subState in"=w37, "menu (get)"=enum16{"set", "get"}."set", "Loop ID"=w93) -> ()  [unwired: 4 in, 4 out]
  n142 = local read "Exit Value"() -> (w92:i32)
  n143 = Bundle By Name(cluster=T5 {"State"=enum."null", "Waiting Loop"=0, "State to Wait For"=0, "Loop ID"=0, "Exit Value"=0, "Joystick Y"=0.0, "Joystick Z"=0.0} ("Loop 2 Data"), "Joystick Y"=w42, "Joystick Z"=w41, "Loop ID"=w94, "Exit Value"=w95, "State"=w36) -> (→"Loop 2 Data":T5)
  n144 = Bundle By Name(cluster=T3 {"State"=enum."null", "Waiting Loop"=0, "State to Wait For"=0, "Loop ID"=0, "Exit Value"=0, "Joystick Y"=0.0, "Tune Setpoint"={"Increment"=FALSE, "Decrement"=FALSE}} ("Loop 3 Data"), "Joystick Y"=w39, "Loop ID"=w93, "Exit Value"=w92, "State"=w37, "Tune Setpoint"=w38) -> (→"Loop 3 Data":T3)
  "Exit Value" <- -1 ("Exit Value")
